vi "Convert To JSON Comp Format.vi"(11 "input settings":T2={"PDM clock rate"=51200.0, "decimation factor"=1, "bit clock direction"=enum."In", "logic level"=enum."3.3 V"} {"decimation factor" items=["24"=24, "32"=32, "48"=48, "64"=64, "96"=96, "128"=128]; "PDM clock rate" format="%#_6p"}) -> (3 "input settings JSON":cluster{"PDM":T1} {"PDM"."PDM clock rate" format="%#_6p"})   [LabVIEW 2022 SP3, in "PDM input cfg file.lvlib"]
uses:
  PDM input cfg file.lvlib
  controls/PDM/PDM input settings.ctl
  <vilib>/PDM Acquisition Toolkit/shared/controls/decimation order.ctl
  controls/bit clock direction.ctl
  <vilib>/PDM Acquisition Toolkit/host/Classes/Session/Controls/Logic Levels.ctl
  controls/PDM/PDM input settings_json.ctl
  <vilib>/PDM Acquisition Toolkit/host/Classes/Session/DecoderSession.lvclass
  <vilib>/PDM Acquisition Toolkit/shared/PDM Shared.lvlib
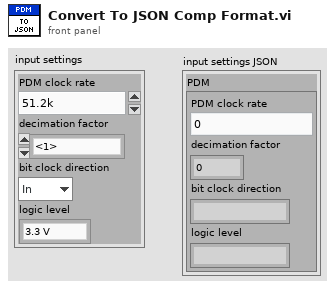
[diagram p1: front panel]
types:
  T1 = typedef "PDM input settings_json.ctl" = cluster{"PDM clock rate":dbl, "decimation factor":dbl, "bit clock direction":string, "logic level":string}
  T2 = typedef "PDM input settings.ctl" = cluster{"PDM clock rate":dbl, "decimation factor":T3, "bit clock direction":T4, "logic level":T5}
  T3 = typedef "PDM Shared.lvlib/decimation order.ctl" = u16
  T4 = typedef "bit clock direction.ctl" = enum32{"In", "Out"}
  T5 = typedef "PDM Acquisition Class Library.lvlib/DecoderSession.lvclass/Logic Levels.ctl" = enum16{"3.3 V", "1.8 V", "1.2 V"}
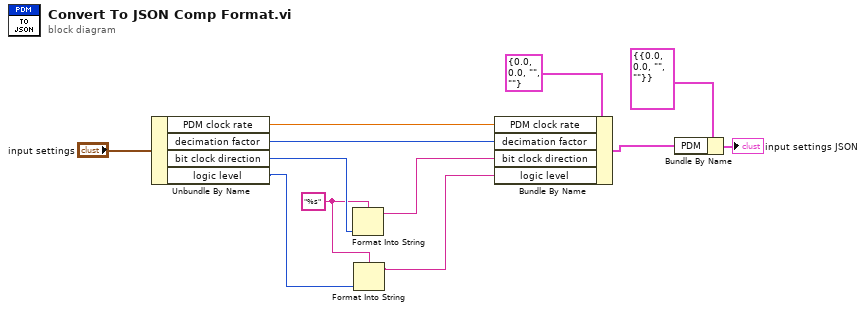
[diagram p0: block diagram]
diagram:
  w4 = "%s" ("format string")
  n1 = Unbundle By Name("input settings") -> ("PDM clock rate"=w7:dbl, "decimation factor"=w8:T3, "bit clock direction"=w11:T4, "logic level"=w5:T5)
  n2 = Format Into String(format string=w4, w11) -> (resulting string=w6:string)  [unwired: 2 in, 1 out]
  n3 = Format Into String(format string=w4, w5) -> (resulting string=w3:string)  [unwired: 2 in, 1 out]
  n4 = Bundle By Name(cluster=T1 {"PDM clock rate"=0.0, "decimation factor"=0.0, "bit clock direction"="", "logic level"=""} ("JSON compatible settings"), "PDM clock rate"=w7, "decimation factor"=w8, "bit clock direction"=w6, "logic level"=w3) -> (w2:T1)
  n5 = Bundle By Name(cluster=cluster{"PDM":T1} {"PDM"={"PDM clock rate"=0.0, "decimation factor"=0.0, "bit clock direction"="", "logic level"=""}}, "PDM"=w2) -> (→"input settings JSON":cluster{"PDM":T1})
